vi "space_vector_algorithm.vi"() -> ()   [LabVIEW 2010]
uses:
  common/classes/SpaceVector/SpaceVector/SpaceVector.lvclass
panel:
  out "no. of points":i32
  out "XY Graph":cluster{dbl[], dbl[]}[](graph)
  in  "kappa":i32=10
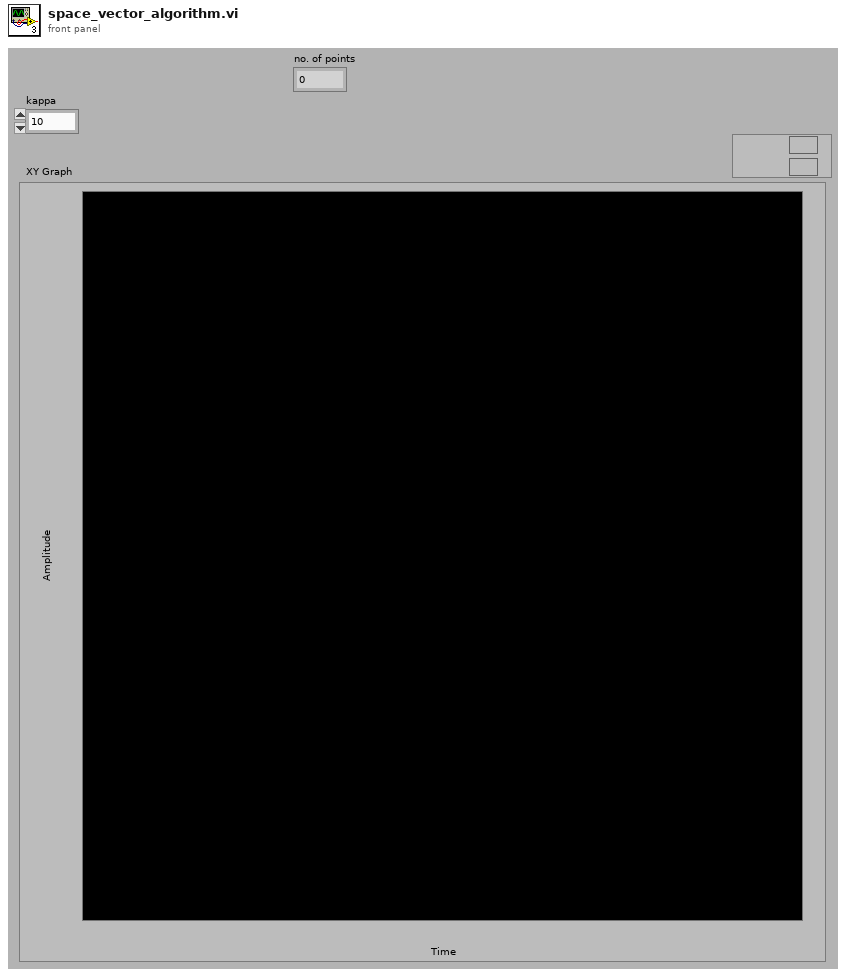
[diagram p1: front panel]
types:
  T1 = cluster{refnum<class "SpaceVector.lvclass">[], refnum<class "SpaceVector.lvclass">[]}
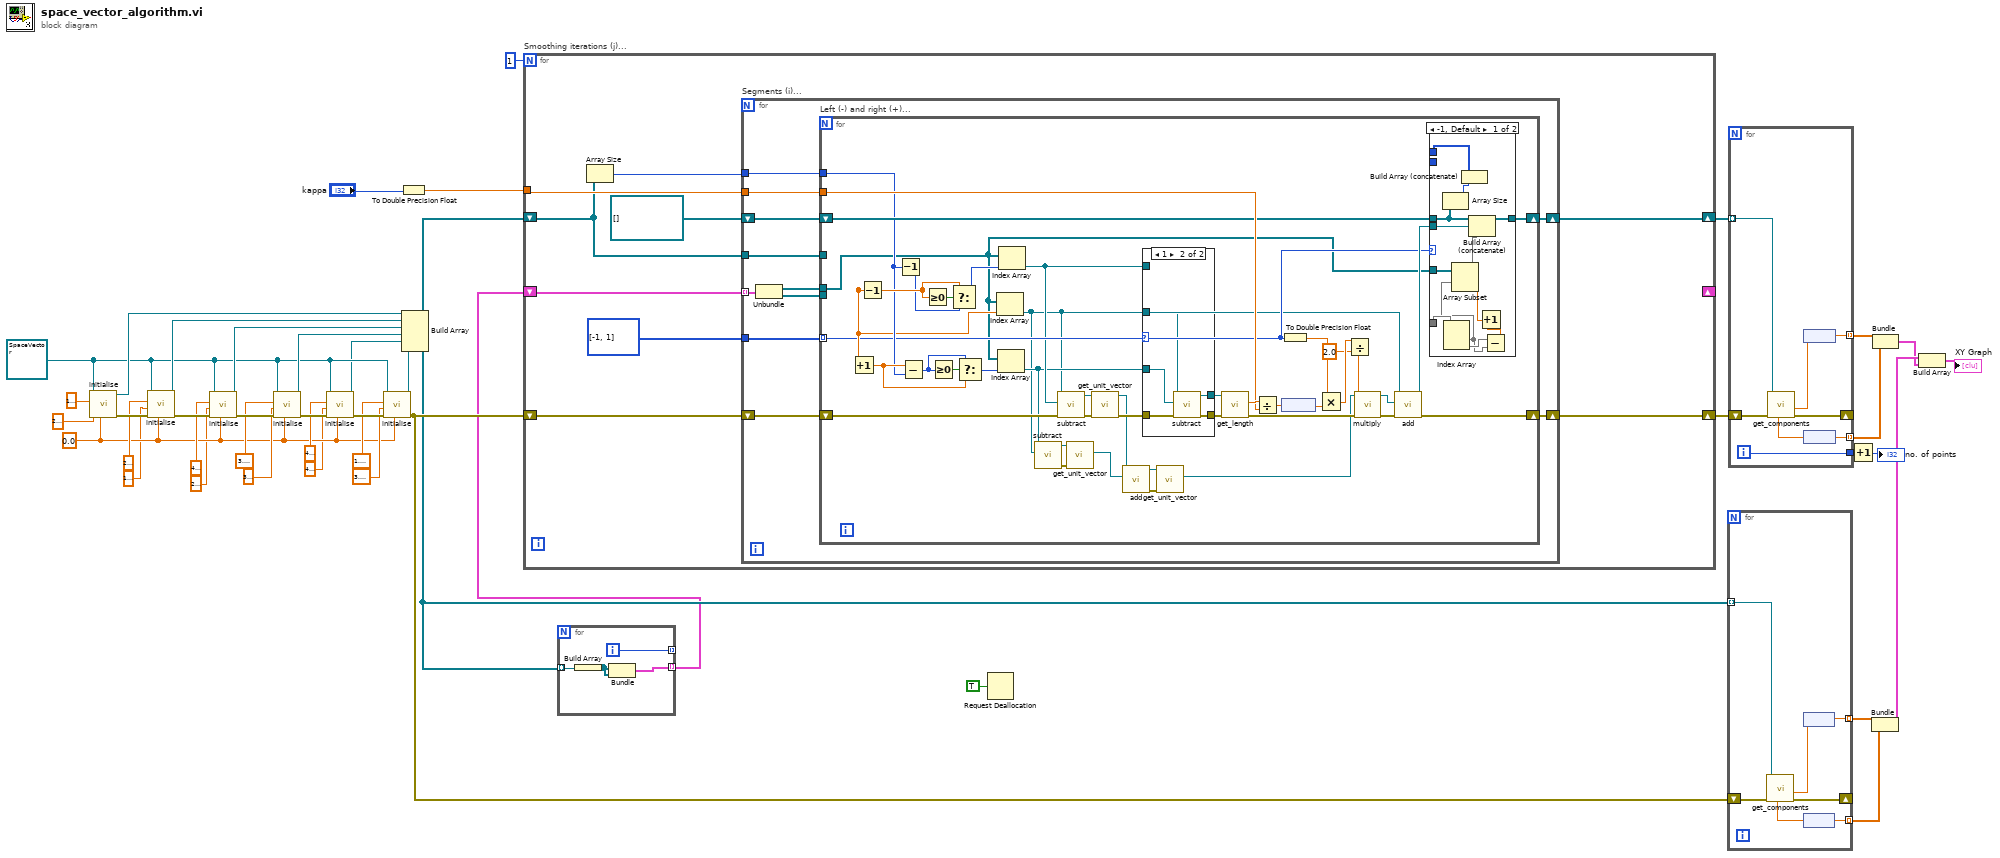
[diagram p0: block diagram]
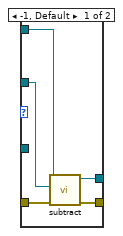
[diagram p2: hidden frame]
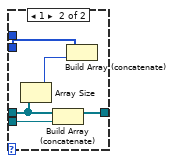
[diagram p3: hidden frame]
diagram:
  w19 = dbl[unit] 0.0 ("z")
  w30 = refnum<class "SpaceVector.lvclass"> refnum ("SpaceVector.lvclass")
  n1 = call "initialise.vi"("z"=w19, "y"=dbl[unit] 2e-06, "x"=dbl[unit] 1e-06, "SpaceVector in"=w30) -> ("error out"=w42:errorcluster, "SpaceVector out"=w38:refnum<class "SpaceVector.lvclass">)  [unwired: 6 in]
  n2 = call "initialise.vi"("z"=w19, "error in (no error)"=w42, "y"=dbl[unit] 1e-06, "x"=dbl[unit] 2e-06, "SpaceVector in"=w30) -> ("error out"=w41:errorcluster, "SpaceVector out"=w37:refnum<class "SpaceVector.lvclass">)  [unwired: 5 in]
  n3 = call "initialise.vi"("z"=w19, "error in (no error)"=w41, "y"=dbl[unit] 2e-06, "x"=dbl[unit] 4e-06, "SpaceVector in"=w30) -> ("error out"=w40:errorcluster, "SpaceVector out"=w36:refnum<class "SpaceVector.lvclass">)  [unwired: 5 in]
  n4 = call "initialise.vi"("z"=w19, "error in (no error)"=w40, "y"=dbl[unit] 3e-06, "x"=dbl[unit] 3.5e-06, "SpaceVector in"=w30) -> ("error out"=w39:errorcluster, "SpaceVector out"=w35:refnum<class "SpaceVector.lvclass">)  [unwired: 5 in]
  n5 = call "initialise.vi"("z"=w19, "error in (no error)"=w39, "y"=dbl[unit] 4.9999999999999996e-06, "x"=dbl[unit] 4e-06, "SpaceVector in"=w30) -> ("error out"=w29:errorcluster, "SpaceVector out"=w28:refnum<class "SpaceVector.lvclass">)  [unwired: 5 in]
  n6 = call "initialise.vi"("z"=w19, "error in (no error)"=w29, "y"=dbl[unit] 3.5e-06, "x"=dbl[unit] 1.5e-06, "SpaceVector in"=w30) -> ("error out"=w10:errorcluster, "SpaceVector out"=w27:refnum<class "SpaceVector.lvclass">)  [unwired: 5 in]
  n7 = To Double Precision Float(number="kappa") -> (double precision float=w34:dbl)
  n8 = Build Array(w38, w37, w36, w35, w28, w27) -> (w4:refnum<class "SpaceVector.lvclass">[])
  n9 = for {
    tunnel: w4 -> [w47] mode=indexing
    tunnel: [w46] -> w1 mode=indexing
    tunnel: [w45] -> _ mode=indexing
    i -> [w45]
    n10 = Build Array(w47) -> (w44:refnum<class "SpaceVector.lvclass">[])
    n11 = Bundle(w44, w44) -> (w46:T1)  [unwired: 1 in]
  }
  n12 = for "Smoothing iterations (j)..." {
    N: 1 -> [_]
    tunnel: w34 -> [w56]
    shift-right: [w52] -> w33
    shift-left: w4 -> [w49]
    shift-right: [w54] -> w32
    shift-left: w10 -> [w55]
    shift-right: _ -> [_]
    shift-left: w1 -> [w48]
    n13 = Array Size(array=w49) -> (size(s)=w51:i32)
    n14 = for "Segments (i)..." {
      tunnel: w56 -> [w67]
      tunnel: w51 -> [w62]
      shift-right: [w65] -> w54
      shift-left: w55 -> [w66]
      tunnel: i32[] [-1, 1] -> [w61]
      shift-right: [w63] -> w52
      shift-left: refnum<class "SpaceVector.lvclass">[] [] -> [w64]
      tunnel: w49 -> [w60]
      tunnel: w48 -> [w59] mode=indexing
      n15 = Unbundle(w59) -> (w58:refnum<class "SpaceVector.lvclass">[], w57:refnum<class "SpaceVector.lvclass">[])
      n16 = for "Left (-) and right (+)..." {
        shift-right: [w86] -> w65
        shift-left: w66 -> [w100]
        tunnel: w67 -> [w105]
        shift-right: [w92] -> w63
        shift-left: w64 -> [w91]
        tunnel: w62 -> [w89]
        tunnel: w61 -> [w82] mode=indexing
        tunnel: w60 -> [_]
        tunnel: w58 -> [w68]
        tunnel: w57 -> [_]
        n17 = Decrement() -> (x=w83:dbl, x-1=w90:dbl)
        n18 = Increment(x=w83) -> (x+1=w95:dbl)
        n19 = Decrement(x=w89) -> (x-1=w88:i32)
        n20 = Subtract(x=w95, y=w89) -> (x-y=w97:i32)
        n21 = Greater Or Equal To 0?(x=w90) -> (x >= 0?=w98:bool)
        n22 = Greater Or Equal To 0?(x=w97) -> (x >= 0?=w96:bool)
        n23 = Select(t=w90, s=w98, f=w88) -> (s? t:f=w87:i32)
        n24 = Select(t=w97, s=w96, f=w95) -> (s? t:f=w94:i32)
        n25 = Index Array(array=w68, index=w83) -> (element=w76:refnum<class "SpaceVector.lvclass">)
        n26 = Index Array(array=w68, index=w94) -> (element=w77:refnum<class "SpaceVector.lvclass">)
        n27 = Index Array(array=w68, index=w87) -> (element=w78:refnum<class "SpaceVector.lvclass">)
        n28 = call "subtract.vi"("subtrahend"=w76, "SpaceVector in"=w77) -> ("error out"=w75:errorcluster, "SpaceVector out"=w74:refnum<class "SpaceVector.lvclass">)  [unwired: 8 in]
        n29 = call "subtract.vi"("error in (no error)"=w100, "subtrahend"=w78, "SpaceVector in"=w76) -> ("error out"=w109:errorcluster, "SpaceVector out"=w110:refnum<class "SpaceVector.lvclass">)  [unwired: 7 in]
        n30 = call "get_unit_vector.vi"("error in (no error)"=w75, "SpaceVector in"=w74) -> ("unit vector"=w72:refnum<class "SpaceVector.lvclass">)  [unwired: 7 in, 2 out]
        n31 = call "get_unit_vector.vi"("error in (no error)"=w109, "SpaceVector in"=w110) -> ("error out"=w101:errorcluster, "SpaceVector out"=w73:refnum<class "SpaceVector.lvclass">)  [unwired: 7 in, 1 out]
        n32 = call "add.vi"("vector to be added"=w72, "SpaceVector in"=w73) -> ("error out"=w71:errorcluster, "SpaceVector out"=w70:refnum<class "SpaceVector.lvclass">)  [unwired: 8 in]
        n33 = case shown="1" w82 {
          tunnel: [w112 w120] -> w108
          tunnel: [w113 w119] -> w107
          tunnel: w101 -> [w111 w118]
          tunnel: w78 -> [w115 _]
          tunnel: w76 -> [w114 w117]
          tunnel: w77 -> [_ w116]
          frame -1, Default {
            n34 = call "subtract.vi"("error in (no error)"=w111, "subtrahend"=w114, "SpaceVector in"=w115) -> ("error out"=w112:errorcluster, "SpaceVector out"=w113:refnum<class "SpaceVector.lvclass">)  [unwired: 7 in]
          }
          frame 1 {
            n35 = call "subtract.vi"("error in (no error)"=w118, "subtrahend"=w116, "SpaceVector in"=w117) -> ("error out"=w120:errorcluster, "SpaceVector out"=w119:refnum<class "SpaceVector.lvclass">)  [unwired: 7 in]
          }
        }
        n36 = call "get_unit_vector.vi"("error in (no error)"=w71, "SpaceVector in"=w70) -> ("unit vector"=w69:refnum<class "SpaceVector.lvclass">)  [unwired: 7 in, 2 out]
        n37 = call "get_length.vi"("error in (no error)"=w108, "SpaceVector in"=w107) -> ("error out"=w99:errorcluster, "length"=w106:dbl[unit])  [unwired: 7 in, 1 out]
        n38 = Divide(x=w106, y=w105) -> (x/y=w104:dbl[unit])
        n39 = node(w104) -> (w85:dbl)
        n40 = To Double Precision Float(number=w82) -> (double precision float=w84:dbl)
        n41 = Multiply(x=w84, y=w85) -> (x*y=w81:dbl)
        n42 = Divide(x=w81, y=2.0) -> (x/y=w79:dbl)
        n43 = call "multiply.vi"("error in (no error)"=w99, "factor"=w79, "SpaceVector in"=w69) -> ("error out"=w103:errorcluster, "SpaceVector out"=w102:refnum<class "SpaceVector.lvclass">)  [unwired: 7 in]
        n44 = call "add.vi"("error in (no error)"=w103, "vector to be added"=w102, "SpaceVector in"=w76) -> ("error out"=w86:errorcluster, "SpaceVector out"=w93:refnum<class "SpaceVector.lvclass">)  [unwired: 7 in]
        n45 = case shown="-1, Default" w82 {
          tunnel: w93 -> [w133 w136]
          tunnel: [w134 w140] -> w92
          tunnel: w91 -> [w129 w137]
          tunnel: _ -> [w131 w139]
          tunnel: _ -> [w132 w138]
          tunnel: w68 -> [w127 _]
          tunnel: _ -> [w125 _]
          frame -1, Default {
            n46 = Array Size(array=w129) -> (size(s)=w128:i32)
            n47 = Index Array(array=w125) -> (element #1=w121, element #2=w123)  [unwired: 2 in]
            n48 = Build Array (concatenate)(w131, w128) -> (w130:i32[])
            n49 = Subtract(x=w123, y=w121) -> (x-y=w122:dbl)
            n50 = Increment(x=w122) -> (x+1=w124:dbl)
            n51 = Array Subset(array=w127, index=w121, length=w124) -> (w126:refnum<class "SpaceVector.lvclass">[])
            n52 = Build Array (concatenate)(w129, w133, w126) -> (w134:refnum<class "SpaceVector.lvclass">[])
          }
          frame 1 {
            n53 = Array Size(array=w137) -> (size(s)=w135:i32)
            n54 = Build Array (concatenate)(w137, w136) -> (w140:refnum<class "SpaceVector.lvclass">[])
            n55 = Build Array (concatenate)(w138, w135) -> ()  [unwired: 1 out]
          }
        }
      }
    }
  }
  n56 = Request Deallocation(TRUE ("flag")) -> ()
  n57 = for {
    tunnel: w4 -> [w146] mode=indexing
    shift-right: [w145] -> _
    shift-left: w10 -> [w147]
    tunnel: [w143] -> w12 mode=indexing
    tunnel: [w141] -> w13 mode=indexing
    n58 = call "get_components.vi"("error in (no error)"=w147, "SpaceVector in"=w146) -> ("error out"=w145:errorcluster, "x"=w144:dbl[unit], "y"=w142:dbl[unit])  [unwired: 4 in, 3 out]
    n59 = node(w144) -> (w143:dbl)
    n60 = node(w142) -> (w141:dbl)
  }
  n61 = for {
    tunnel: w33 -> [w154] mode=indexing
    shift-right: [w153] -> _
    shift-left: w32 -> [w155]
    tunnel: [w151] -> w31 mode=indexing
    tunnel: [w149] -> w14 mode=indexing
    tunnel: [w148] -> w8
    i -> [w148]
    n62 = call "get_components.vi"("error in (no error)"=w155, "SpaceVector in"=w154) -> ("error out"=w153:errorcluster, "x"=w152:dbl[unit], "y"=w150:dbl[unit])  [unwired: 4 in, 3 out]
    n63 = node(w152) -> (w151:dbl)
    n64 = node(w150) -> (w149:dbl)
  }
  n65 = Increment(x=w8) -> (x+1=→"no. of points":i32)
  n66 = Bundle(w12, w13) -> (w6:cluster{dbl[], dbl[]})  [unwired: 1 in]
  n67 = Bundle(w31, w14) -> (w5:cluster{dbl[], dbl[]})  [unwired: 1 in]
  n68 = Build Array(w6, w5) -> (→"XY Graph":cluster{dbl[], dbl[]}[])
